vi "pH meter.vi"() -> ()   [LabVIEW 2012]
doc: "This update adds the license features. It does not make any other significant changes."
uses:
  DAQ configuration/channel identifier.ctl
  TCP DAQ/Sensor data.ctl
  DAQ configuration/sensor cluster.ctl
  toolbar icons/log data.ctl
  toolbar icons/gran.ctl
  calibration/pH/pH Gran plot.ctl
  calibration/pH/pH gran type.ctl
  toolbar icons/save gran.ctl
  calibration/calib array.ctl
  calibration/conversion.ctl
  DAQ configuration/scale type.ctl
  calibration/correspondence table.ctl
  calibration/pH/pH scale.ctl
  calibration/Dissolved Oxygen/DO scale.ctl
  calibration/pH/pH titration.ctl
  toolbar icons/data not logging.ctl
  toolbar icons/Data Source.ctl
  toolbar icons/help.ctl
  calibration/global scale array.vi
panel:
  in  "Help Button":T1
  in  "change Va":bool
  in  "Temperature cal":T2={"conversion matrix"=[[20.13986, 0.0], [100.6023, 1.0]], "units"="deg C", "name"="Temperature", "scale type"=enum."Polynomial", "offset (volts)"=0.0, "second channel"=-1, "correspondence table"=[], "offset (physical units)"=0.0, "pH scale"={"Buffers"=[], "Temperature"=0.0}, "D.O."={"Temperature"=0.0, "K"=0.0, "barometric pressure"=0.0}} {"D.O."."K" format="%.6f"; "D.O."."Temperature" format="%.2f"; "pH scale"."Buffers"."V/T" format="%.5f"; "pH scale"."Buffers"."Buffer" format="%.2f"; "pH scale"."Temperature" format="%.2f"; "offset (physical units)" format="%.5f"; "correspondence table"."volts" format="%.4f"; "correspondence table"."physical units" format="%.4f"; "second channel" min=-1; "offset (volts)" format="%.5f"; "conversion matrix" format="%.4e"}
  in  "data server address":string="dataserver.cee.cornell.edu"
  in  "Data Source":T7 caption="OK Button"
  in  "Temperature":dbl[unit]=293.15 format="%.1f"
  in  "Temperature\ncompensated":bool=TRUE
  in  "File Comment":bool
  out "File path":path
  out "file warning":T8
  in  "connection ID":refnum<k5>
  out "incremental titrant added":dbl format="%.3f"
  out "Titrating":bool
  out "Titration":T9 {"Nt" format="%.4f"; "Vo" format="%.3f"}
  out "Temperature Location":string
  out "pH location":string
  in  "default cal":T11=[{"conversion matrix"=[[0.0, 0.0], [0.0, 0.0], [0.0, 0.0], [0.0, 0.0], [0.0, 0.0], [0.0, 0.0]], "units"="pH", "name"="pH", "scale type"=enum."pH", "offset (volts)"=0.0, "second channel"=1, "correspondence table"=[], "offset (physical units)"=0.0, "pH scale"={"Buffers"=[{"Buffer"=4.0, "Calibrated"=FALSE, "V/T"=0.0013599919516459151}, {"Buffer"=7.0, "Calibrated"=FALSE, "V/T"=0.0}, {"Buffer"=10.0, "Calibrated"=FALSE, "V/T"=0.0}], "Temperature"=20.0}, "D.O."={"Temperature"=0.0, "K"=0.0, "barometric pressure"=0.0}}, {"conversion matrix"=[[20.13986, 0.0], [100.6023, 1.0]], "units"="deg C", "name"="Temperature", "scale type"=enum."Polynomial", "offset (volts)"=0.0, "second channel"=-1, "correspondence table"=[], "offset (physical units)"=0.0, "pH scale"={"Buffers"=[], "Temperature"=0.0}, "D.O."={"Temperature"=0.0, "K"=0.0, "barometric pressure"=0.0}}] {"D.O."."K" format="%.6f"; "D.O."."Temperature" format="%.2f"; "pH scale"."Buffers"."V/T" format="%.5f"; "pH scale"."Buffers"."Buffer" format="%.2f"; "pH scale"."Temperature" format="%.2f"; "offset (physical units)" format="%.5f"; "correspondence table"."volts" format="%.4f"; "correspondence table"."physical units" format="%.4f"; "second channel" min=-1; "offset (volts)" format="%.5f"; "conversion matrix" format="%.4e"}
  in  "Save Gran Plot":T12
  in  "End Titration":bool
  in  "accept pH value":bool
  out "Gran Plot":T13={"Ve"=0.5, "ANC"=0.5, "r"=0.5, "Gran type"=enum."ANC", "Gran Plot"=[], "pH"=[]} {"r" format="%.4f"; "ANC" format="%.2p"; "Ve" format="%.3f"; "pH" format="%.2f"}
  in  "Edit buffers":bool
  out "Buffers":T14(array[cluster]) {"V/T" format="%.2f"; "Buffer" format="%.2f"}
  in  "Gran Plot":T15
  out "File ref":refnum<file>
  in  "Data log file":T16
  in  "index":enum16{"pH", "Temperature"}(ring)
  out "Sample Temperature":dbl[unit] format="%.2f"
  out "pH voltage":sgl format="%.2f"
  in  "Data interval (s)":ext=1.0 format="%.3f"
  out "Sensor Data":T17 {"Sensor array"."scaled" format="%.2f"; "Sensor array"."voltage" format="%.4f"; "Time" format="%<%I:%M:%S%2u %p\n%m/%d/%Y>T"}
  out "pH":dbl format="%.3f"
  in  "Sensor Array":i32[](array[numeric])
  in  "Clear buffers":bool
  in  "Add buffer":bool
  in  "Temperature":T19 items=["SC1Mod1/ai0", "SC1Mod1/ai1", "SC1Mod1/ai2", "SC1Mod1/ai3", "SC1Mod1/ai4", "SC1Mod1/ai5", "SC1Mod1/ai6", "SC1Mod1/ai7", "SC1Mod1/ai8", "SC1Mod1/ai9", "SC1Mod1/ai10", "SC1Mod1/ai11", "SC1Mod1/ai12", "SC1Mod1/ai13", "SC1Mod1/ai14", "SC1Mod1/ai15", "SC1Mod1/ai16", "SC1Mod1/ai17", "SC1Mod1/ai18", "SC1Mod1/ai19", "SC1Mod1/ai20", "SC1Mod1/ai21", "SC1Mod1/ai22", "SC1Mod1/ai23", "SC1Mod1/ai24", "SC1Mod1/ai25", "SC1Mod1/ai26", "SC1Mod1/ai27", "SC1Mod1/ai28", "SC1Mod1/ai29", "SC1Mod1/ai30", "SC1Mod1/ai31", "SC1Mod2/ai0", "SC1Mod2/ai1", "SC1Mod2/ai2", "SC1Mod2/ai3", "SC1Mod2/ai4", "SC1Mod2/ai5", "SC1Mod2/ai6", "SC1Mod2/ai7", "SC1Mod2/ai8", "SC1Mod2/ai9", "SC1Mod2/ai10", "SC1Mod2/ai11", "SC1Mod2/ai12", "SC1Mod2/ai13", "SC1Mod2/ai14", "SC1Mod2/ai15", "SC1Mod2/ai16", "SC1Mod2/ai17", "SC1Mod2/ai18", "SC1Mod2/ai19", "SC1Mod2/ai20", "SC1Mod2/ai21", "SC1Mod2/ai22", "SC1Mod2/ai23", "SC1Mod2/ai24", "SC1Mod2/ai25", "SC1Mod2/ai26", "SC1Mod2/ai27", "SC1Mod2/ai28", "SC1Mod2/ai29", "SC1Mod2/ai30", "SC1Mod2/ai31", "SC1Mod3/ai0", "SC1Mod3/ai1", "SC1Mod3/ai2", "SC1Mod3/ai3", "SC1Mod3/ai4", "SC1Mod3/ai5", "SC1Mod3/ai6", "SC1Mod3/ai7", "SC1Mod3/ai8", "SC1Mod3/ai9", "SC1Mod3/ai10", "SC1Mod3/ai11", "SC1Mod3/ai12", "SC1Mod3/ai13", "SC1Mod3/ai14", "SC1Mod3/ai15", "SC1Mod3/ai16", "SC1Mod3/ai17", "SC1Mod3/ai18", "SC1Mod3/ai19", "SC1Mod3/ai20", "SC1Mod3/ai21", "SC1Mod3/ai22", "SC1Mod3/ai23", "SC1Mod3/ai24", "SC1Mod3/ai25", "SC1Mod3/ai26", "SC1Mod3/ai27", "SC1Mod3/ai28", "SC1Mod3/ai29", "SC1Mod3/ai30", "SC1Mod3/ai31", "SC1Mod4/ai0", "SC1Mod4/ai1", "SC1Mod4/ai2", "SC1Mod4/ai3", "SC1Mod4/ai4", "SC1Mod4/ai5", "SC1Mod4/ai6", "SC1Mod4/ai7", "SC1Mod4/ai8", "SC1Mod4/ai9", "SC1Mod4/ai10", "SC1Mod4/ai11", "SC1Mod4/ai12", "SC1Mod4/ai13", "SC1Mod4/ai14", "SC1Mod4/ai15", "SC1Mod4/ai16", "SC1Mod4/ai17", "SC1Mod4/ai18", "SC1Mod4/ai19", "SC1Mod4/ai20", "SC1Mod4/ai21", "SC1Mod4/ai22", "SC1Mod4/ai23", "SC1Mod4/ai24", "SC1Mod4/ai25", "SC1Mod4/ai26", "SC1Mod4/ai27", "SC1Mod4/ai28", "SC1Mod4/ai29", "SC1Mod4/ai30", "SC1Mod4/ai31"]
  in  "pH probe":T19 items=["SC1Mod1/ai0", "SC1Mod1/ai1", "SC1Mod1/ai2", "SC1Mod1/ai3", "SC1Mod1/ai4", "SC1Mod1/ai5", "SC1Mod1/ai6", "SC1Mod1/ai7", "SC1Mod1/ai8", "SC1Mod1/ai9", "SC1Mod1/ai10", "SC1Mod1/ai11", "SC1Mod1/ai12", "SC1Mod1/ai13", "SC1Mod1/ai14", "SC1Mod1/ai15", "SC1Mod1/ai16", "SC1Mod1/ai17", "SC1Mod1/ai18", "SC1Mod1/ai19", "SC1Mod1/ai20", "SC1Mod1/ai21", "SC1Mod1/ai22", "SC1Mod1/ai23", "SC1Mod1/ai24", "SC1Mod1/ai25", "SC1Mod1/ai26", "SC1Mod1/ai27", "SC1Mod1/ai28", "SC1Mod1/ai29", "SC1Mod1/ai30", "SC1Mod1/ai31", "SC1Mod2/ai0", "SC1Mod2/ai1", "SC1Mod2/ai2", "SC1Mod2/ai3", "SC1Mod2/ai4", "SC1Mod2/ai5", "SC1Mod2/ai6", "SC1Mod2/ai7", "SC1Mod2/ai8", "SC1Mod2/ai9", "SC1Mod2/ai10", "SC1Mod2/ai11", "SC1Mod2/ai12", "SC1Mod2/ai13", "SC1Mod2/ai14", "SC1Mod2/ai15", "SC1Mod2/ai16", "SC1Mod2/ai17", "SC1Mod2/ai18", "SC1Mod2/ai19", "SC1Mod2/ai20", "SC1Mod2/ai21", "SC1Mod2/ai22", "SC1Mod2/ai23", "SC1Mod2/ai24", "SC1Mod2/ai25", "SC1Mod2/ai26", "SC1Mod2/ai27", "SC1Mod2/ai28", "SC1Mod2/ai29", "SC1Mod2/ai30", "SC1Mod2/ai31", "SC1Mod3/ai0", "SC1Mod3/ai1", "SC1Mod3/ai2", "SC1Mod3/ai3", "SC1Mod3/ai4", "SC1Mod3/ai5", "SC1Mod3/ai6", "SC1Mod3/ai7", "SC1Mod3/ai8", "SC1Mod3/ai9", "SC1Mod3/ai10", "SC1Mod3/ai11", "SC1Mod3/ai12", "SC1Mod3/ai13", "SC1Mod3/ai14", "SC1Mod3/ai15", "SC1Mod3/ai16", "SC1Mod3/ai17", "SC1Mod3/ai18", "SC1Mod3/ai19", "SC1Mod3/ai20", "SC1Mod3/ai21", "SC1Mod3/ai22", "SC1Mod3/ai23", "SC1Mod3/ai24", "SC1Mod3/ai25", "SC1Mod3/ai26", "SC1Mod3/ai27", "SC1Mod3/ai28", "SC1Mod3/ai29", "SC1Mod3/ai30", "SC1Mod3/ai31", "SC1Mod4/ai0", "SC1Mod4/ai1", "SC1Mod4/ai2", "SC1Mod4/ai3", "SC1Mod4/ai4", "SC1Mod4/ai5", "SC1Mod4/ai6", "SC1Mod4/ai7", "SC1Mod4/ai8", "SC1Mod4/ai9", "SC1Mod4/ai10", "SC1Mod4/ai11", "SC1Mod4/ai12", "SC1Mod4/ai13", "SC1Mod4/ai14", "SC1Mod4/ai15", "SC1Mod4/ai16", "SC1Mod4/ai17", "SC1Mod4/ai18", "SC1Mod4/ai19", "SC1Mod4/ai20", "SC1Mod4/ai21", "SC1Mod4/ai22", "SC1Mod4/ai23", "SC1Mod4/ai24", "SC1Mod4/ai25", "SC1Mod4/ai26", "SC1Mod4/ai27", "SC1Mod4/ai28", "SC1Mod4/ai29", "SC1Mod4/ai30", "SC1Mod4/ai31"]
  out "Quit":bool
  in  "Clear graph":bool
  in  "history length":u16=1000
  out "XY Graph":cluster{dbl[], dbl[]}[](graph)
  # "C"
  # "kPa"
  # "C"
  # "Normality of titrant"
  # "eq/L"
  # "mL"
  # "Volume of sample"
  # "C"
  # "kPa"
  # "C"
  # "mL"
  # "eq/L"
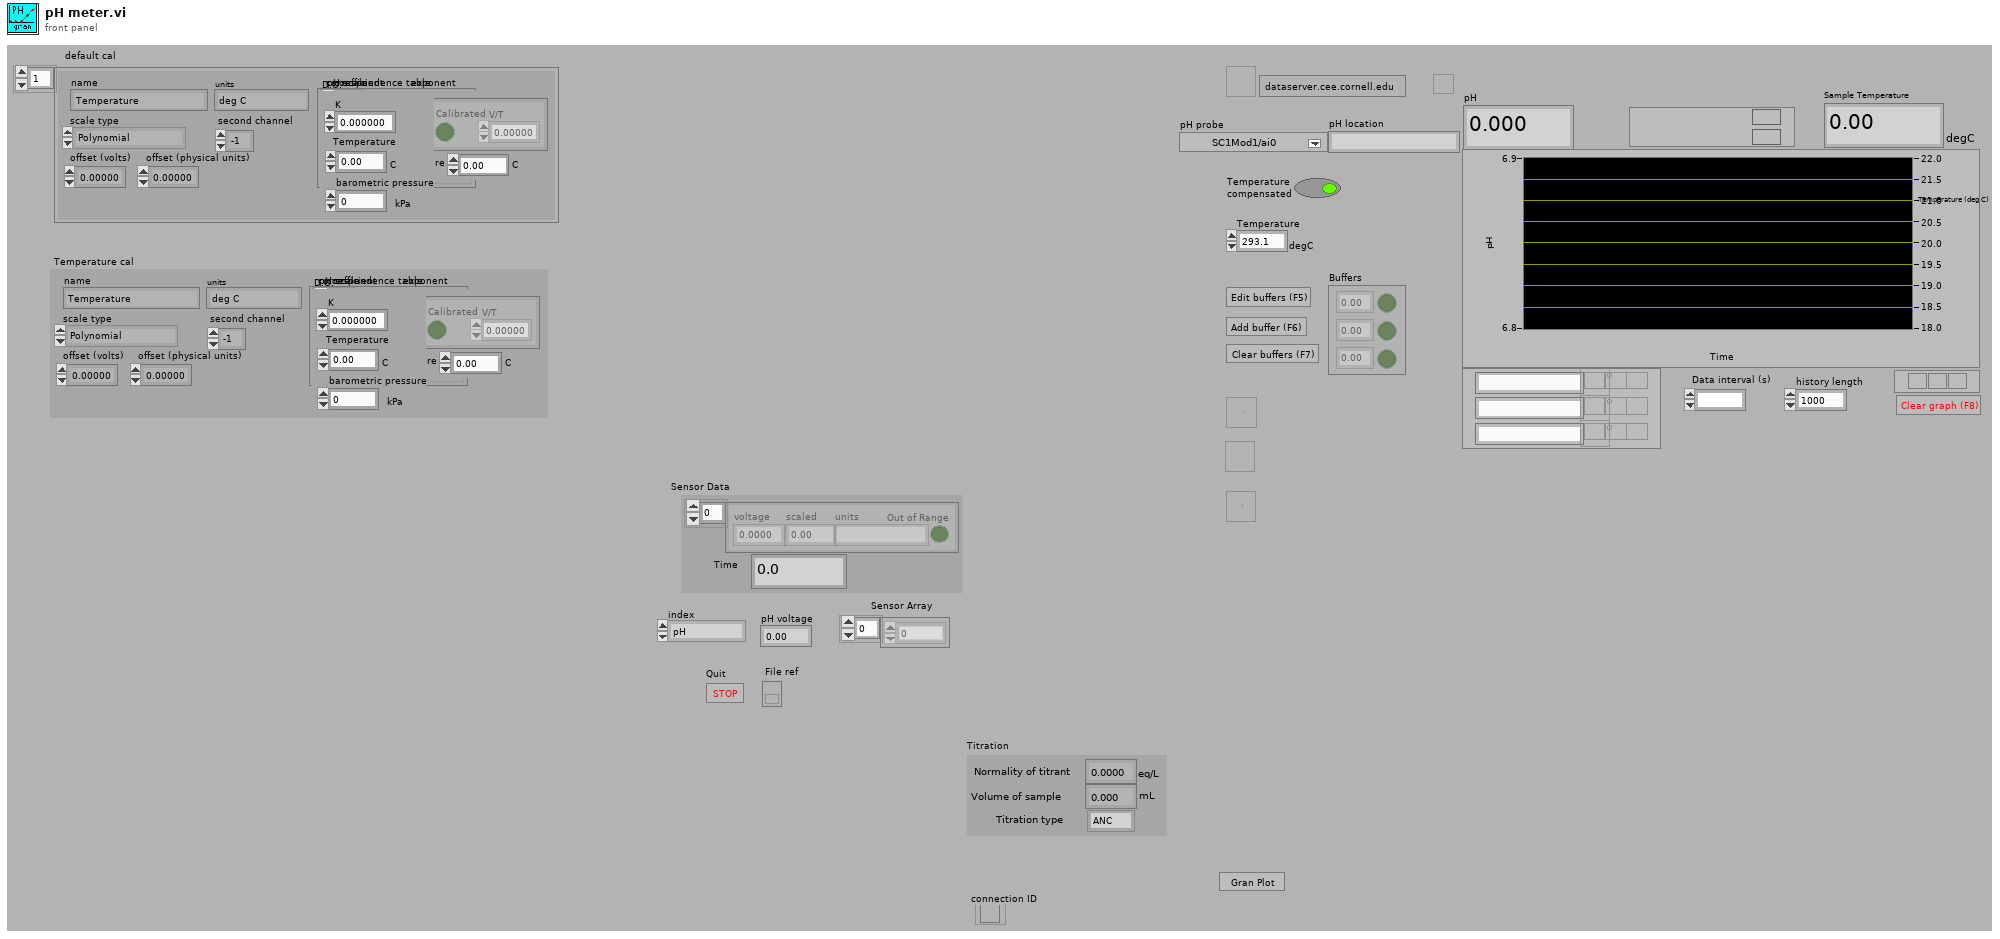
[diagram p1: front panel]
types:
  T1 = typedef "help.ctl" = bool
  T2 = typedef "conversion.ctl" = cluster{"conversion matrix":sgl[][], "units":string, "name":string, "scale type":T3, "offset (volts)":dbl, "second channel":i8, "correspondence table":T4, "offset (physical units)":dbl, "pH scale":T5, "D.O.":T6}
  T3 = typedef "scale type.ctl" = enum16{"Volts", "Polynomial", "Correspondence Table", "pH", "Dissolved Oxygen", "Quadratic"}
  T4 = typedef "correspondence table.ctl" = cluster{"physical units":dbl, "volts":dbl}[]
  T5 = typedef "pH scale.ctl" = cluster{"Buffers":cluster{"Buffer":dbl, "Calibrated":bool, "V/T":dbl}[], "Temperature":dbl}
  T6 = typedef "DO scale.ctl" = cluster{"Temperature":dbl, "K":dbl, "barometric pressure":dbl}
  T7 = typedef "Data Source.ctl" = bool
  T8 = typedef "data not logging.ctl" = bool
  T9 = typedef "pH titration.ctl" = cluster{"Vo":dbl, "Nt":dbl, "Titration type":T10}
  T10 = typedef "pH gran type.ctl" = enum16{"ANC", "BNC"}
  T11 = typedef "calib array.ctl" = T2[]
  T12 = typedef "save gran.ctl" = bool
  T13 = typedef "pH Gran plot.ctl" = cluster{"Ve":dbl, "ANC":dbl, "r":dbl, "Gran type":T10, "Gran Plot":cluster{"Va":dbl[], "F1":dbl[]}[], "pH":dbl[]}
  T14 = cluster{"Buffer":dbl, "Calibrated":bool, "V/T":dbl}[]
  T15 = typedef "gran.ctl" = bool
  T16 = typedef "log data.ctl" = bool
  T17 = typedef "Sensor data.ctl" = cluster{" Sensor array":T18[], "Time":dbl}
  T18 = typedef "sensor cluster.ctl" = cluster{"voltage":sgl, "scaled":sgl, "units":string, "Out of Range":bool}
  T19 = typedef "channel identifier.ctl" = u16
  T20 = typedef "Server stats.ctl" = cluster{"scan rate":dbl, "# connections":i32, "channel settings":cluster{"Name":string, "upper input limits":sgl, "lower input limits":sgl, "Location":string}[]}
  T21 = cluster{"Name":string, "upper input limits":sgl, "lower input limits":sgl, "Location":string}[]
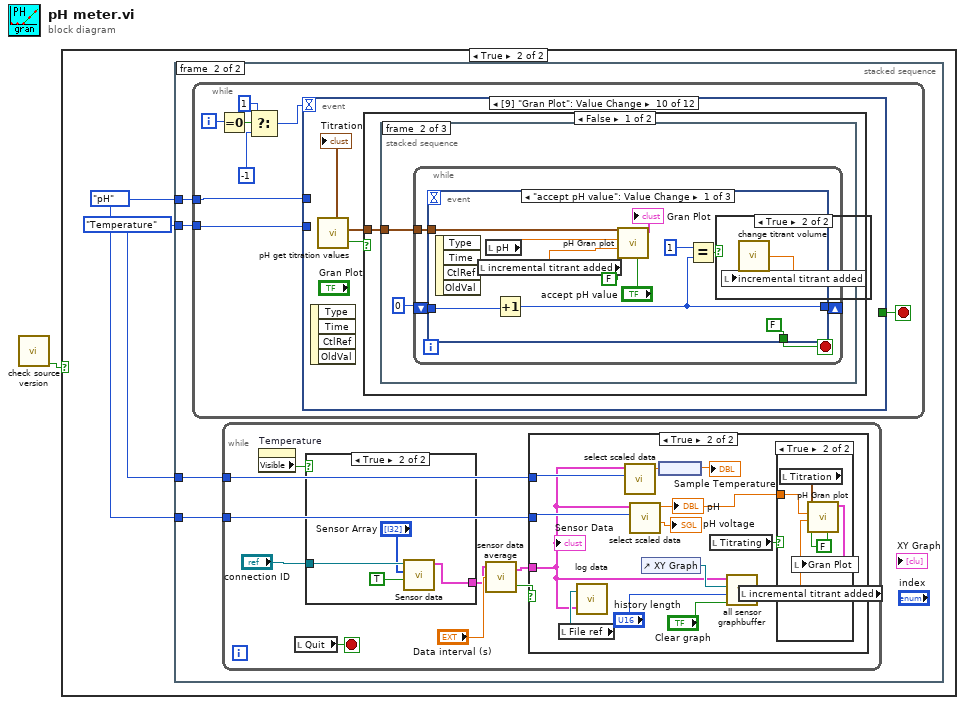
[diagram p0: block diagram]
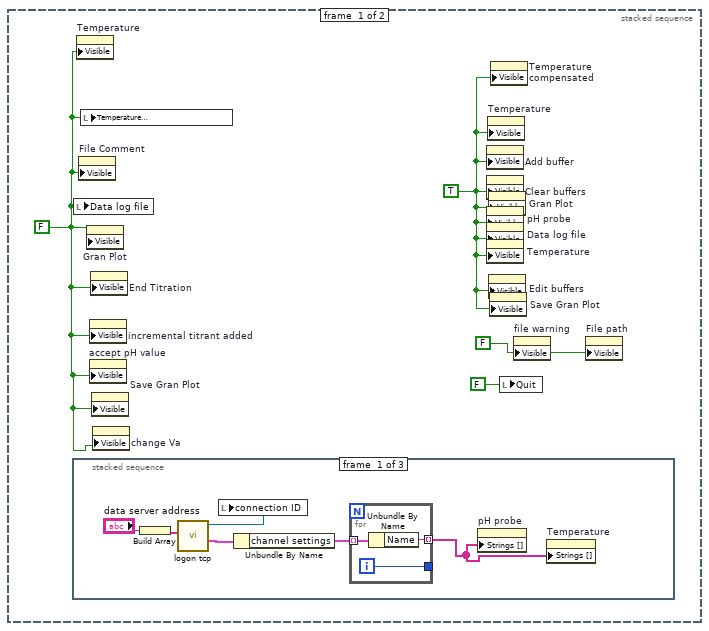
[diagram p3: hidden frame]
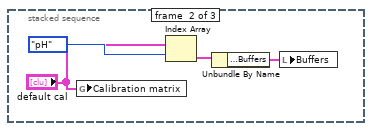
[diagram p4: hidden frame]
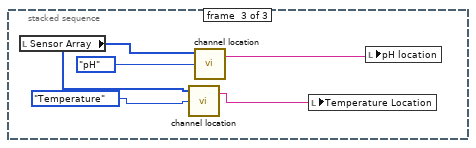
[diagram p5: hidden frame]
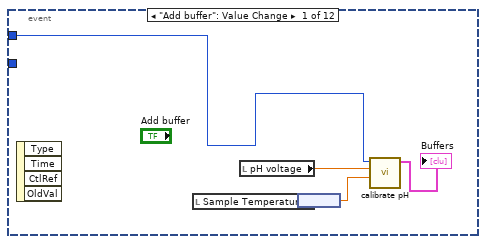
[diagram p6: hidden frame]
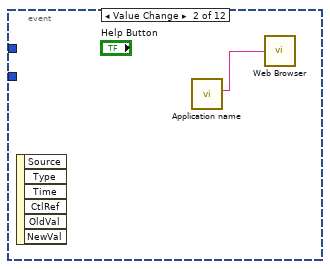
[diagram p7: hidden frame]
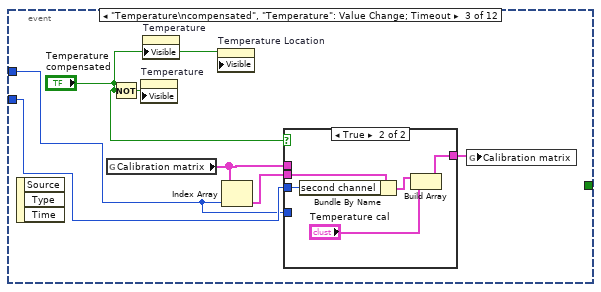
[diagram p8: hidden frame]
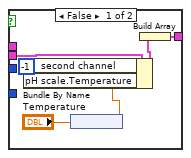
[diagram p9: hidden frame]
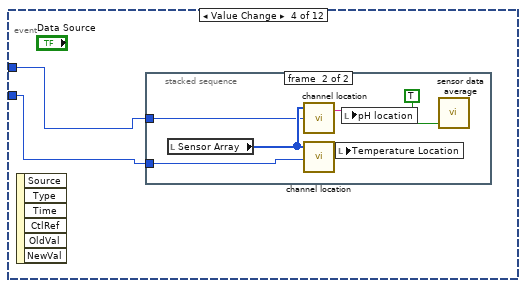
[diagram p10: hidden frame]
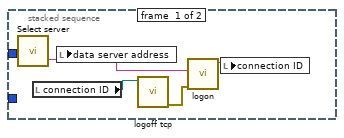
[diagram p11: hidden frame]
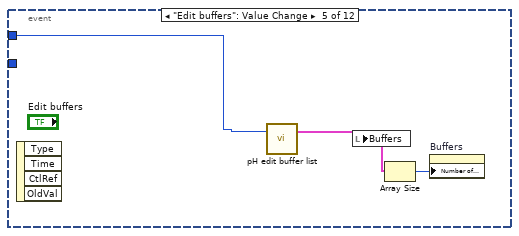
[diagram p12: hidden frame]
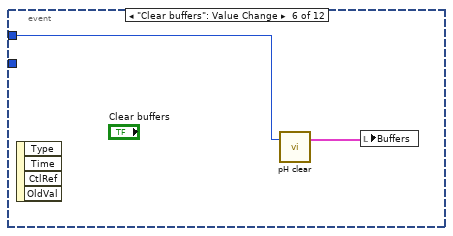
[diagram p13: hidden frame]
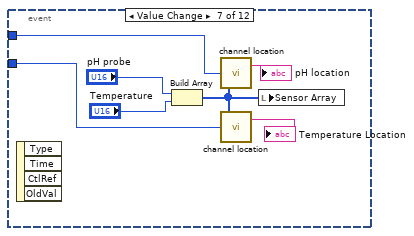
[diagram p14: hidden frame]
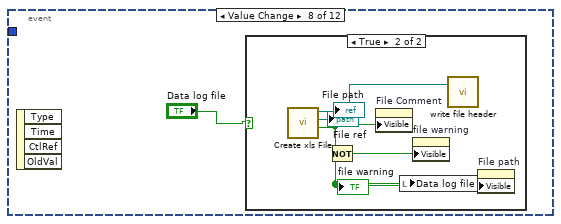
[diagram p15: hidden frame]
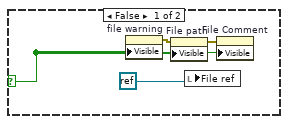
[diagram p16: hidden frame]
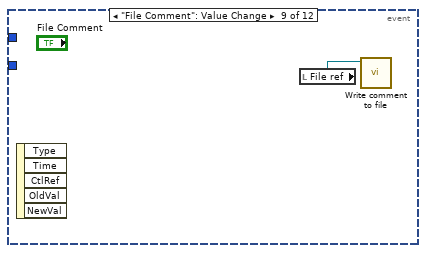
[diagram p17: hidden frame]
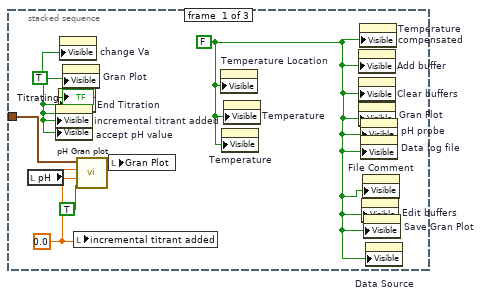
[diagram p18: hidden frame]
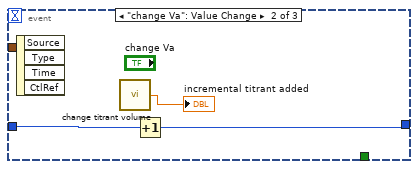
[diagram p20: hidden frame]
diagram:
  n1 = call "check source version.vi"() -> ("continue running?"=w1:bool)  [unwired: 2 in, 3 out]
  n2 = case shown="True" w1 {
    frame False {
    }
    frame True {
      w2 = enum16{"pH", "Temperature"}."Temperature" ("index")
      w3 = enum16{"pH", "Temperature"}."pH" ("index")
      n3 = stacked-sequence {
        tunnel: w3 -> [_ w29]
        tunnel: w2 -> [_ w28]
        tunnel: w2 -> [_ w27]
        tunnel: w3 -> [_ w26]
        frame #0 {
          w4 = TRUE ("Visible")
          w5 = FALSE ("Visible")
          w6 = FALSE ("File Failure")
          n4 = stacked-sequence {
            frame #0 {
              n5 = Build Array("data server address") -> (w11:string[])
              n6 = call "logon tcp.vi"("Data Servers"=w11) -> ("Server stats"=w10:T20, "connection ID"=w13:refnum<k5>)  [unwired: 5 in, 4 out]
              n7 = local write "connection ID"(w13) -> ()
              n8 = Unbundle By Name(w10) -> ("channel settings"=w9:T21)
              n9 = for {
                tunnel: w9 -> [w16] mode=indexing
                tunnel: [w15] -> w8 mode=indexing
                tunnel: [w14] -> _
                i -> [w14]
                n10 = Unbundle By Name(w16) -> ("Name"=w15:string)
              }
              n11 = property on="pH probe" class="Ring (strict)"("Strings []"=w8) -> ()  [unwired: 2 in, 2 out]
              n12 = property on="Temperature" class="Ring (strict)"("Strings []"=w8) -> ()  [unwired: 2 in, 2 out]
            }
            frame #1 {
              n13 = global write "global scale array.vi" "Calibration matrix"("default cal") -> ()
              n14 = Index Array(array="default cal", index=enum16{"pH", "Temperature"}."pH") -> (element=w18:T2)
              n15 = Unbundle By Name(w18) -> ("pH scale.Buffers"=w19:T14)
              n16 = local write "Buffers"(w19) -> ()
            }
            frame #2 {
              n17 = local read "Sensor Array"() -> (w23:i32[])
              n18 = call "channel location.vi"("Index"=enum16{"pH", "Temperature"}."Temperature" ("index"), "Sensor Array"=w23) -> ("Port Location"=w21:string)  [unwired: 2 in]
              n19 = call "channel location.vi"("Index"=enum16{"pH", "Temperature"}."pH" ("index"), "Sensor Array"=w23) -> ("Port Location"=w24:string)  [unwired: 2 in]
              n20 = local write "Temperature Location"(w21) -> ()
              n21 = local write "pH location"(w24) -> ()
            }
          }
          n22 = local write "Data log file"(w5) -> ()
          n23 = property on="Temperature" class="Ring (strict)"("Visible"=w5) -> ()  [unwired: 2 in, 2 out]
          n24 = property on="File Comment" class="Bool"("Visible"=w5) -> ()  [unwired: 2 in, 2 out]
          n25 = local write "Temperature\ncompensated"(w5) -> ()
          n26 = property on="Gran Plot" class="Clust (strict)"("Visible"=w5) -> ()  [unwired: 2 in, 2 out]
          n27 = property on="incremental titrant added" class="DigNum (strict)"("Visible"=w5) -> ()  [unwired: 2 in, 2 out]
          n28 = property on="accept pH value" class="Bool"("Visible"=w5) -> ()  [unwired: 2 in, 2 out]
          n29 = property on="End Titration" class="Bool"("Visible"=w5) -> ()  [unwired: 2 in, 2 out]
          n30 = property on="Save Gran Plot" class="Bool"("Visible"=w5) -> ()  [unwired: 2 in, 2 out]
          n31 = property on="change Va" class="Bool"("Visible"=w5) -> ()  [unwired: 2 in, 2 out]
          n32 = property on="Add buffer" class="Bool"("Visible"=w4) -> ()  [unwired: 2 in, 2 out]
          n33 = property on="Clear buffers" class="Bool"("Visible"=w4) -> ()  [unwired: 2 in, 2 out]
          n34 = property on="pH probe" class="Ring (strict)"("Visible"=w4) -> ()  [unwired: 2 in, 2 out]
          n35 = property on="Data log file" class="Bool (strict)"("Visible"=w4) -> ()  [unwired: 2 in, 2 out]
          n36 = property on="Temperature" class="Ring (strict)"("Visible"=w4) -> ()  [unwired: 2 in, 2 out]
          n37 = property on="Temperature" class="DigNum (strict)"("Visible"=w4) -> ()  [unwired: 2 in, 2 out]
          n38 = property on="Gran Plot" class="Bool"("Visible"=w4) -> ()  [unwired: 2 in, 2 out]
          n39 = property on="Edit buffers" class="Bool"("Visible"=w4) -> ()  [unwired: 2 in, 2 out]
          n40 = property on="Save Gran Plot" class="Bool"("Visible"=w4) -> ()  [unwired: 2 in, 2 out]
          n41 = property on="Temperature\ncompensated" class="Bool (strict)"("Visible"=w4) -> ()  [unwired: 2 in, 2 out]
          n42 = local write "Quit"(FALSE ("Quit")) -> ()
          n43 = property on="file warning" class="Bool"("Visible"=w6) -> ()  [unwired: 2 in, 2 out]
          n44 = property on="File path" class="Path"("Visible"=w6) -> ()  [unwired: 2 in, 2 out]
        }
        frame #1 {
          n45 = while {
            tunnel: w29 -> [w36]
            tunnel: w28 -> [w35]
            i -> [w34]
            stop <- w37 stop-if-true
            n46 = Equal To 0?(x=w34) -> (x = 0?=w33:bool)
            n47 = Select(t=1, s=w33, f=-1) -> (s? t:f=w30:i32)
            n48 = event shown="[9] \"Gran Plot\": Value Change" {
              selector: _ -> [_ _ _ _ _ _ _ _ _ _ _ _]
              dyn-events: _ -> [_ _ _ _ _ _ _ _ _ _ _ _]
              timeout: w30 -> [_ _ _ _ _ _ _ _ _ _ _ _]
              tunnel: [_ _ _ _ _ _ _ _ _ _ _ w167] -> w37
              tunnel: w36 -> [w39 _ w46 w63 w74 w77 w84 _ _ _ _ _]
              tunnel: w35 -> [_ _ w48 w62 _ _ w81 _ _ _ _ _]
              event "Add buffer": Value Change {
                n49 = event-data() -> ()  [unwired: 1 in, 4 out]
                n50 = local read "Sample Temperature"() -> (w42:dbl[unit])
                n51 = local read "pH voltage"() -> (w41:sgl)
                n52 = node(w42) -> (w40:dbl)
                n53 = call "calibrate pH.vi"("index"=w39, "pH voltage"=w41, "Temperature"=w40) -> ("Buffers"=→"Buffers":T14)  [unwired: 7 in]
              }
              event Value Change {
                n54 = event-data() -> ()  [unwired: 1 in, 6 out]
                n55 = call "Application name.vi"() -> ("help site"=w43:string)  [unwired: 5 in, 2 out]
                n56 = call "Web Browser.vi"("URL"=w43) -> ()  [unwired: 1 in]
              }
              event "Temperature\ncompensated", "Temperature": Value Change; Timeout {
                n57 = event-data() -> ()  [unwired: 1 in, 3 out]
                n58 = global read "global scale array.vi" "Calibration matrix"() -> (w47:T11)
                n59 = Not(x="Temperature\ncompensated") -> (.not. x?=w50:bool)
                n60 = property on="Temperature" class="DigNum (strict)"("Visible"=w50) -> ()  [unwired: 2 in, 2 out]
                n61 = property on="Temperature" class="Ring (strict)"("Visible"="Temperature\ncompensated") -> ()  [unwired: 2 in, 2 out]
                n62 = property on="Temperature Location" class="Str"("Visible"="Temperature\ncompensated") -> ()  [unwired: 2 in, 2 out]
                n63 = Index Array(array=w47, index=w46) -> (element=w49:T2)
                n64 = case shown="True" "Temperature\ncompensated" {
                  tunnel: w49 -> [w56 w61]
                  tunnel: w48 -> [_ w60]
                  tunnel: w47 -> [_ _]
                  tunnel: w46 -> [_ _]
                  tunnel: [w53 w58] -> w45
                  frame False {
                    n65 = node("Temperature") -> (w51:dbl)
                    n66 = Bundle By Name(cluster=w56, "second channel"=i8 -1, "pH scale.Temperature"=w51) -> (w54:T2)
                    n67 = Build Array(w54) -> (w53:T2[])
                  }
                  frame True {
                    n68 = Bundle By Name(cluster=w61, "second channel"=w60) -> (w59:T2)
                    n69 = Build Array(w59, "Temperature cal") -> (w58:T2[])
                  }
                }
                n70 = global write "global scale array.vi" "Calibration matrix"(w45) -> ()
              }
              event Value Change {
                n71 = event-data() -> ()  [unwired: 1 in, 6 out]
                n72 = stacked-sequence {
                  tunnel: w63 -> [_ w71]
                  tunnel: w62 -> [_ w70]
                  frame #0 {
                    n73 = call "Select server.vi"() -> ("DataSource"=w67:string)  [unwired: 5 in]
                    n74 = local read "connection ID"() -> (w65:refnum<k5>)
                    n75 = local write "data server address"(w67) -> ()
                    n76 = call "logoff tcp.vi"("Connection ID"=w65) -> ("error out"=w64:errorcluster)  [unwired: 9 in, 1 out]
                    n77 = call "logon.vi"("error in"=w64, "data server address in"=w67) -> ("connection ID"=w66:refnum<k5>)  [unwired: 6 in, 3 out]
                    n78 = local write "connection ID"(w66) -> ()
                  }
                  frame #1 {
                    n79 = local read "Sensor Array"() -> (w72:i32[])
                    n80 = call "channel location.vi"("Index"=w71, "Sensor Array"=w72) -> ("Port Location"=w69:string)  [unwired: 2 in]
                    n81 = call "channel location.vi"("Index"=w70, "Sensor Array"=w72) -> ("Port Location"=w73:string)  [unwired: 2 in]
                    n82 = local write "Temperature Location"(w73) -> ()
                    n83 = local write "pH location"(w69) -> ()
                    n84 = call "sensor data average.vi"("Reset"=TRUE) -> ()  [unwired: 2 in, 2 out]
                  }
                }
              }
              event "Edit buffers": Value Change {
                n85 = event-data() -> ()  [unwired: 1 in, 4 out]
                n86 = call "pH edit buffer list.vi"("index"=w74) -> ("Buffers out"=w75:T14)  [unwired: 2 in]
                n87 = local write "Buffers"(w75) -> ()
                n88 = Array Size(array=w75) -> (size(s)=w76:i32)
                n89 = property on="Buffers" class="Arr (strict)"("Number of Rows"=w76) -> ()  [unwired: 2 in, 2 out]
              }
              event "Clear buffers": Value Change {
                n90 = event-data() -> ()  [unwired: 1 in, 4 out]
                n91 = call "pH clear.vi"("index"=w77) -> ("Buffers"=w78:T14)  [unwired: 2 in]
                n92 = local write "Buffers"(w78) -> ()
              }
              event Value Change {
                n93 = event-data() -> ()  [unwired: 1 in, 4 out]
                n94 = Build Array("pH probe", "Temperature") -> (w80:T19[])
                n95 = call "channel location.vi"("Index"=w84, "Sensor Array"=w80) -> ("Port Location"=→"pH location":string)  [unwired: 2 in]
                n96 = call "channel location.vi"("Index"=w81, "Sensor Array"=w80) -> ("Port Location"=→"Temperature Location":string)  [unwired: 2 in]
                n97 = local write "Sensor Array"(w80) -> ()
              }
              event Value Change {
                n98 = event-data() -> ()  [unwired: 1 in, 4 out]
                n99 = case shown="True" "Data log file" {
                  selector: "Data log file" -> [w89 _]
                  frame False {
                    n100 = property on="file warning" class="Bool"("Visible"=w89) -> (error out=w87:errorcluster)  [unwired: 2 in, 1 out]
                    n101 = property on="File path" class="Path"(error in=w87, "Visible"=w89) -> (error out=w88:errorcluster)  [unwired: 1 in, 1 out]
                    n102 = local write "File ref"(refnum<k0> refnum) -> ()
                    n103 = property on="File Comment" class="Bool"(error in=w88, "Visible"=w89) -> ()  [unwired: 1 in, 2 out]
                  }
                  frame True {
                    n104 = call "Create xls File.vi"() -> ("Valid File"=w91:bool, "path"=→"File path":path, "refnum"=w94:refnum<file>)  [unwired: 4 in, 1 out]
                    "File ref" <- w94
                    "file warning" <- w91
                    n105 = Not(x=w91) -> (.not. x?=w93:bool)
                    n106 = property on="File Comment" class="Bool"("Visible"=w91) -> ()  [unwired: 2 in, 2 out]
                    n107 = local write "Data log file"(w91) -> ()
                    n108 = property on="file warning" class="Bool"("Visible"=w93) -> ()  [unwired: 2 in, 2 out]
                    n109 = call "write file header.vi"("refnum"=w94) -> ()  [unwired: 2 in, 1 out]
                    n110 = property on="File path" class="Path"("Visible"=w91) -> ()  [unwired: 2 in, 2 out]
                  }
                }
              }
              event "File Comment": Value Change {
                n111 = event-data() -> ()  [unwired: 1 in, 5 out]
                n112 = local read "File ref"() -> (w95:refnum<file>)
                n113 = call "Write comment to file.vi"("refnum"=w95) -> ()  [unwired: 7 in, 2 out]
              }
              event Value Change {
                n114 = event-data() -> ()  [unwired: 1 in, 4 out]
                n115 = call "pH get titration values.vi"() -> ("canceled"=w96:bool, "Titration"=w97:T9)  [unwired: 2 in]
                "Titration" <- w97
                n116 = case shown="False" w96 {
                  tunnel: w97 -> [w98 _]
                  frame False {
                    n117 = stacked-sequence {
                      tunnel: w98 -> [w102 w107 _]
                      frame #0 {
                        w101 = 0.0 ("incremental titrant added")
                        w99 = TRUE ("Visible")
                        w100 = FALSE ("Visible")
                        n118 = local read "pH"() -> (w104:dbl)
                        n119 = property on="incremental titrant added" class="DigNum (strict)"("Visible"=w99) -> ()  [unwired: 2 in, 2 out]
                        n120 = property on="accept pH value" class="Bool"("Visible"=w99) -> ()  [unwired: 2 in, 2 out]
                        n121 = property on="End Titration" class="Bool"("Visible"=w99) -> ()  [unwired: 2 in, 2 out]
                        n122 = property on="change Va" class="Bool"("Visible"=w99) -> ()  [unwired: 2 in, 2 out]
                        n123 = property on="Gran Plot" class="Clust (strict)"("Visible"=w99) -> ()  [unwired: 2 in, 2 out]
                        n124 = local write "incremental titrant added"(w101) -> ()
                        n125 = call "pH Gran plot.vi"("initialize"=TRUE, "amount of titrant added"=w101, "pH"=w104, "sample"=w102) -> ("Gran plot"=w105:T13)  [unwired: 7 in]
                        n126 = local write "Gran Plot"(w105) -> ()
                        n127 = property on="Temperature Location" class="Str"("Visible"=w100) -> ()  [unwired: 2 in, 2 out]
                        n128 = property on="Temperature" class="Ring (strict)"("Visible"=w100) -> ()  [unwired: 2 in, 2 out]
                        n129 = property on="Temperature" class="DigNum (strict)"("Visible"=w100) -> ()  [unwired: 2 in, 2 out]
                        n130 = property on="Add buffer" class="Bool"("Visible"=w100) -> ()  [unwired: 2 in, 2 out]
                        n131 = property on="Clear buffers" class="Bool"("Visible"=w100) -> ()  [unwired: 2 in, 2 out]
                        n132 = property on="Gran Plot" class="Bool"("Visible"=w100) -> ()  [unwired: 2 in, 2 out]
                        n133 = property on="Temperature\ncompensated" class="Bool (strict)"("Visible"=w100) -> ()  [unwired: 2 in, 2 out]
                        n134 = property on="pH probe" class="Ring (strict)"("Visible"=w100) -> ()  [unwired: 2 in, 2 out]
                        n135 = property on="Data log file" class="Bool (strict)"("Visible"=w100) -> ()  [unwired: 2 in, 2 out]
                        n136 = property on="Edit buffers" class="Bool"("Visible"=w100) -> ()  [unwired: 2 in, 2 out]
                        n137 = property on="File Comment" class="Bool"("Visible"=w100) -> ()  [unwired: 2 in, 2 out]
                        n138 = property on="Save Gran Plot" class="Bool"("Visible"=w100) -> ()  [unwired: 2 in, 2 out]
                        n139 = property on="Data Source" class="Bool"("Visible"=w100) -> ()  [unwired: 2 in, 2 out]
                        "Titrating" <- w99
                      }
                      frame #1 {
                        n140 = while {
                          tunnel: w107 -> [w110]
                          shift-right: [w108] -> _
                          shift-left: 0 -> [w109]
                          stop <- w111 stop-if-true
                          n141 = event shown="[0] \"accept pH value\": Value Change" {
                            selector: _ -> [_ _ _]
                            dyn-events: _ -> [_ _ _]
                            timeout: _ -> [_ _ _]
                            tunnel: [FALSE ("End Titration") _ "End Titration"] -> w111
                            tunnel: w110 -> [w122 _ _]
                            tunnel: w109 -> [w115 w125 w127]
                            tunnel: [w113 w124 w127] -> w108
                            event "accept pH value": Value Change {
                              n142 = event-data() -> ()  [unwired: 1 in, 4 out]
                              n143 = local read "incremental titrant added"() -> (w116:dbl)
                              n144 = local read "pH"() -> (w121:dbl)
                              n145 = Increment(x=w115) -> (x+1=w113:i32)
                              n146 = call "pH Gran plot.vi"("accept pH value"="accept pH value", "initialize"=FALSE, "amount of titrant added"=w116, "pH"=w121, "sample"=w122) -> ("Gran plot"=→"Gran Plot":T13)  [unwired: 6 in]
                              n147 = Equal?(x=1, y=w113) -> (x = y?=w114:bool)
                              n148 = case shown="True" w114 {
                                frame False {
                                }
                                frame True {
                                n149 = call "change titrant volume.vi"() -> ("incremental titrant added out"=w123:dbl)  [unwired: 2 in]
                                n150 = local write "incremental titrant added"(w123) -> ()
                                }
                              }
                            }
                            event "change Va": Value Change {
                              n151 = event-data() -> ()  [unwired: 1 in, 4 out]
                              n152 = call "change titrant volume.vi"() -> ("incremental titrant added out"=→"incremental titrant added":dbl)  [unwired: 2 in]
                              n153 = Increment(x=w125) -> (x+1=w124:i32)
                            }
                            event "End Titration": Value Change {
                              n154 = event-data() -> ()  [unwired: 1 in, 4 out]
                            }
                          }
                        }
                      }
                      frame #2 {
                        w129 = FALSE ("Visible")
                        w132 = TRUE ("Visible")
                        n155 = local read "Temperature\ncompensated"() -> (w131:bool)
                        n156 = local read "Data log file"() -> (w133:T16)
                        n157 = local write "Titrating"(w129) -> ()
                        n158 = property on="change Va" class="Bool"("Visible"=w129) -> ()  [unwired: 2 in, 2 out]
                        n159 = property on="incremental titrant added" class="DigNum (strict)"("Visible"=w129) -> ()  [unwired: 2 in, 2 out]
                        n160 = property on="accept pH value" class="Bool"("Visible"=w129) -> ()  [unwired: 2 in, 2 out]
                        n161 = property on="End Titration" class="Bool"("Visible"=w129) -> ()  [unwired: 2 in, 2 out]
                        n162 = property on="File Comment" class="Bool"("Visible"=w133) -> ()  [unwired: 2 in, 2 out]
                        n163 = Not(x=w131) -> (.not. x?=w130:bool)
                        n164 = property on="Temperature" class="DigNum (strict)"("Visible"=w130) -> ()  [unwired: 2 in, 2 out]
                        n165 = property on="Temperature" class="Ring (strict)"("Visible"=w131) -> ()  [unwired: 2 in, 2 out]
                        n166 = property on="Temperature Location" class="Str"("Visible"=w131) -> ()  [unwired: 2 in, 2 out]
                        n167 = property on="Temperature\ncompensated" class="Bool (strict)"("Visible"=w132) -> ()  [unwired: 2 in, 2 out]
                        n168 = property on="Add buffer" class="Bool"("Visible"=w132) -> ()  [unwired: 2 in, 2 out]
                        n169 = property on="Clear buffers" class="Bool"("Visible"=w132) -> ()  [unwired: 2 in, 2 out]
                        n170 = property on="pH probe" class="Ring (strict)"("Visible"=w132) -> ()  [unwired: 2 in, 2 out]
                        n171 = property on="Data log file" class="Bool (strict)"("Visible"=w132) -> ()  [unwired: 2 in, 2 out]
                        n172 = property on="Gran Plot" class="Bool"("Visible"=w132) -> ()  [unwired: 2 in, 2 out]
                        n173 = property on="Data Source" class="Bool"("Visible"=w132) -> ()  [unwired: 2 in, 2 out]
                        n174 = property on="Edit buffers" class="Bool"("Visible"=w132) -> ()  [unwired: 2 in, 2 out]
                        n175 = property on="Save Gran Plot" class="Bool"("Visible"=w132) -> ()  [unwired: 2 in, 2 out]
                      }
                    }
                  }
                  frame True {
                  }
                }
              }
              event Value Change {
                w143 = "%.8f" ("format (%.3f)")
                n176 = event-data() -> ()  [unwired: 1 in, 5 out]
                n177 = local read "Gran Plot"() -> (w165:T13)
                n178 = local read "Titration"() -> (w141:T9)
                n179 = Unbundle By Name(w165) -> ("Ve"=w156:dbl, "ANC"=w155:dbl, "r"=w154:dbl, "Gran Plot"=w164:cluster{"Va":dbl[], "F1":dbl[]}[], "pH"=w158:dbl[])  [unwired: 1 out]
                n180 = Unbundle By Name(w141) -> ("Vo"=w139:dbl, "Nt"=w140:dbl)
                n181 = Index Array(array=w164, index=0) -> (element=w162:cluster{"Va":dbl[], "F1":dbl[]})
                n182 = Build Array(w139, w140, w156, w155, w154) -> (w136:dbl[])
                n183 = Unbundle By Name(w162) -> ("Va"=w159:dbl[], "F1"=w157:dbl[])
                n184 = Build Array(w159, w158, w157) -> (w145:dbl[][])
                n185 = Build Array("Sample Volume (ml)", "Titrant normality", "Equivalent Volume (ml)", "ANC (eq/L)", "correlation coefficient") -> (w134:string[])
                n186 = Build Array("Titrant Volume (ml)", "pH", "F1") -> (w135:string[])
                n187 = call "Create xls File.vi"() -> ("refnum"=w161:refnum<file>)  [unwired: 4 in, 3 out]
                n188 = call "Write str to xls File.vi"("1D data"=w134, "refnum"=w161) -> ("dup refnum"=w160:refnum<file>)  [unwired: 8 in, 1 out]
                n189 = call "Write to xls File.vi"("format (%.3f)"=w143, "1D data"=w136, "refnum"=w160) -> ("dup refnum"=w150:refnum<file>)  [unwired: 7 in, 1 out]
                n190 = call "Write str to xls File.vi"("1D data"=w135, "refnum"=w150) -> ("dup refnum"=w146:refnum<file>)  [unwired: 8 in, 1 out]
                n191 = call "Write to xls File.vi"("transpose? (no:F)"=TRUE, "format (%.3f)"=w143, "2D data"=w145, "refnum"=w146) -> ("dup refnum"=w142:refnum<file>)  [unwired: 6 in, 1 out]
                n192 = Close File(refnum=w142) -> ()  [unwired: 1 in, 2 out]
              }
              event Application Instance Close? {
                w167 = TRUE ("Quit")
                n193 = event-data() -> ()  [unwired: 1 in, 2 out]
                n194 = local read "connection ID"() -> (w166:refnum<k5>)
                n195 = call "logoff tcp.vi"("Connection ID"=w166) -> ()  [unwired: 9 in, 2 out]
                n196 = event-data() -> ()  [unwired: 2 in, 1 out]
                "Quit" <- w167
              }
            }
          }
          n197 = while {
            tunnel: w27 -> [w172]
            tunnel: w26 -> [w171]
            stop <- w176 stop-if-true
            n198 = property on="Temperature" class="Ring (strict)"() -> ("Visible"=w170:bool)  [unwired: 2 in, 2 out]
            n199 = local read "Quit"() -> (w176:bool)
            n200 = case shown="True" w170 {
              tunnel: "connection ID" -> [w181 w187]
              tunnel: [w178 w185] -> w168
              frame False {
                n201 = local read "pH probe"() -> (w182:T19)
                n202 = local read "Temperature"() -> (w183:dbl[unit])
                n203 = Build Array(w182) -> (w180:T19[])
                n204 = call "Sensor data.vi"("Update channels"=TRUE, "Sensor Array"=w180, "Connection ID in"=w181) -> ("Sensor Data"=w179:T17)  [unwired: 1 in, 7 out]
                n205 = call "Insert temperature.vi"("Temperature"=w183, "Sensor Data"=w179) -> ("Sensor Data out"=w178:T17)
              }
              frame True {
                n206 = call "Sensor data.vi"("Update channels"=TRUE, "Sensor Array"="Sensor Array", "Connection ID in"=w187) -> ("Sensor Data"=w185:T17)  [unwired: 1 in, 7 out]
              }
            }
            n207 = call "sensor data average.vi"("Data interval (s)"="Data interval (s)", "Sensor Data"=w168) -> ("new data"=w173:bool, "Sensor Data out"=w174:T17)  [unwired: 1 in]
            n208 = case shown="True" w173 {
              tunnel: w174 -> [_ w188]
              tunnel: w172 -> [_ w194]
              tunnel: w171 -> [_ w193]
              frame False {
              }
              frame True {
                n209 = local read "File ref"() -> (w196:refnum<file>)
                n210 = call "log data.vi"("Sensor Data"=w188, "refnum"=w196) -> ()  [unwired: 2 in]
                n211 = call "select scaled data.vi"("Sensor index"=w194, "Sensor Data"=w188) -> ("scaled"=w189:sgl)  [unwired: 4 in, 5 out]
                n212 = call "select scaled data.vi"("Sensor index"=w193, "Sensor Data"=w188) -> ("voltage"=→"pH voltage":sgl, "scaled"=w192:sgl)  [unwired: 4 in, 4 out]
                "pH" <- w192
                n213 = control-ref of="XY Graph"() -> (w197:refnum<vi>)
                n214 = node(w189) -> (→"Sample Temperature":sgl[unit])
                n215 = local read "Titrating"() -> (w195:bool)
                n216 = call "all sensor graphbuffer.vi"("Reset"="Clear graph", "history length"="history length", "WFGraph Refnum"=w197, "Sensor Data"=w188) -> ()  [unwired: 5 in, 3 out]
                n217 = case shown="True" w195 {
                  tunnel: w192 -> [_ w203]
                  frame False {
                  }
                  frame True {
                    w200 = FALSE ("accept pH value")
                    n218 = local read "incremental titrant added"() -> (w202:dbl)
                    n219 = local read "Titration"() -> (w204:T9)
                    n220 = call "pH Gran plot.vi"("accept pH value"=w200, "initialize"=w200, "amount of titrant added"=w202, "pH"=w203, "sample"=w204) -> ("Gran plot"=w201:T13)  [unwired: 6 in]
                    n221 = local write "Gran Plot"(w201) -> ()
                  }
                }
                "Sensor Data" <- w188
              }
            }
          }
        }
      }
    }
  }
